vi "Load Settings from XML.vi"(8 "error in (no error)":errorcluster, 11 "Settings in":T1={"Hardware Configuration"={"AI"={"DAQmx Channel"="", "Max Input"=0.0, "Min Input"=0.0, "Sample Rate"=0.0, "DAQmx Task"="", "shunt resistor location"=-1, "external shunt resistor value"=249.0}, "AO"={"DAQmx Channel"="", "Max Output"=0.0, "Min Output"=0.0, "Sample Rate"=0.0, "DAQmx Task"=""}, "DO"={"DAQmx Channel"="", "Sample Rate"=0.0, "DAQmx Task"=""}, "DI"={"DAQmx Channel"="", "Sample Rate"=0.0, "DAQmx Task"=""}, "TC"={"DAQmx Channel"="", "Max Inout"=0.0, "Min Input"=0.0, "Sample Rate"=0.0, "DAQmx Task"="", "resistance configuration"=4, "r0"=100.0, "current excitation value"=0.0025, "current excitation source"=10167, "rtd type"=12481}}, "Logging Configuration"={"Log File Base Path"=path "", "TDMS File Reference"=refnum, "Samples to Save"=0, "Trigger - Time"=0, "Trigger - Threshold"=0.0, "Trigger - Channel"=0, "Enable Time Trigger"=FALSE, "Enable Threshold Trigger"=FALSE, "Always Log"=FALSE}} {"Hardware Configuration"."TC"."rtd type" items=["Pt3750"=12481, "Pt3851"=10071, "Pt3911"=12482, "Pt3916"=10069, "Pt3920"=10053, "Pt3928"=12483, "Custom"=10137]; "Hardware Configuration"."TC"."current excitation source" items=["Internal"=10200, "External"=10167, "None"=10230]; "Hardware Configuration"."TC"."resistance configuration" items=["2-Wire"=2, "3-Wire"=3, "4-Wire"=4]; "Hardware Configuration"."AI"."shunt resistor location" items=["default"=-1, "RSE"=10083, "NRSE"=10078, "Differential"=10106, "Pseudodifferential"=12529]}) -> (0 "error out":errorcluster, 3 "Settings out":T1={"Hardware Configuration"={"AI"={"DAQmx Channel"="", "Max Input"=0.0, "Min Input"=0.0, "Sample Rate"=0.0, "DAQmx Task"="", "shunt resistor location"=-1, "external shunt resistor value"=249.0}, "AO"={"DAQmx Channel"="", "Max Output"=0.0, "Min Output"=0.0, "Sample Rate"=0.0, "DAQmx Task"=""}, "DO"={"DAQmx Channel"="", "Sample Rate"=0.0, "DAQmx Task"=""}, "DI"={"DAQmx Channel"="", "Sample Rate"=0.0, "DAQmx Task"=""}, "TC"={"DAQmx Channel"="", "Max Inout"=0.0, "Min Input"=0.0, "Sample Rate"=0.0, "DAQmx Task"="", "resistance configuration"=4, "r0"=100.0, "current excitation value"=0.0025, "current excitation source"=10167, "rtd type"=12481}}, "Logging Configuration"={"Log File Base Path"=path "", "TDMS File Reference"=refnum, "Samples to Save"=0, "Trigger - Time"=0, "Trigger - Threshold"=0.0, "Trigger - Channel"=0, "Enable Time Trigger"=FALSE, "Enable Threshold Trigger"=FALSE, "Always Log"=FALSE}} {"Hardware Configuration"."TC"."rtd type" items=["Pt3750"=12481, "Pt3851"=10071, "Pt3911"=12482, "Pt3916"=10069, "Pt3920"=10053, "Pt3928"=12483, "Custom"=10137]; "Hardware Configuration"."TC"."current excitation source" items=["Internal"=10200, "External"=10167, "None"=10230]; "Hardware Configuration"."TC"."resistance configuration" items=["2-Wire"=2, "3-Wire"=3, "4-Wire"=4]; "Hardware Configuration"."AI"."shunt resistor location" items=["default"=-1, "RSE"=10083, "NRSE"=10078, "Differential"=10106, "Pseudodifferential"=12529]})   [LabVIEW 2024, in "Settings.lvlib"]
doc: "Attempts to load previous user specified settings from an XML file.\n\nThis VI will not generate an error. If a suitable XML file can't be loaded and parsed then it will simply return the default settings."
uses:
  Settings.lvlib
  Settings.ctl
  Acquisition/Hardware Configuration.ctl
  Logging/Logging Configuration.ctl
  <vilib>/Utility/xml.llb/Read From XML File(string).vi
  <vilib>/Utility/xml.llb/Write to XML File(string).vi
  Acquisition/Acquisition.lvlib
  Logging/Logging.lvlib
panel:
  # "(Scroll up for Settings Controls)"
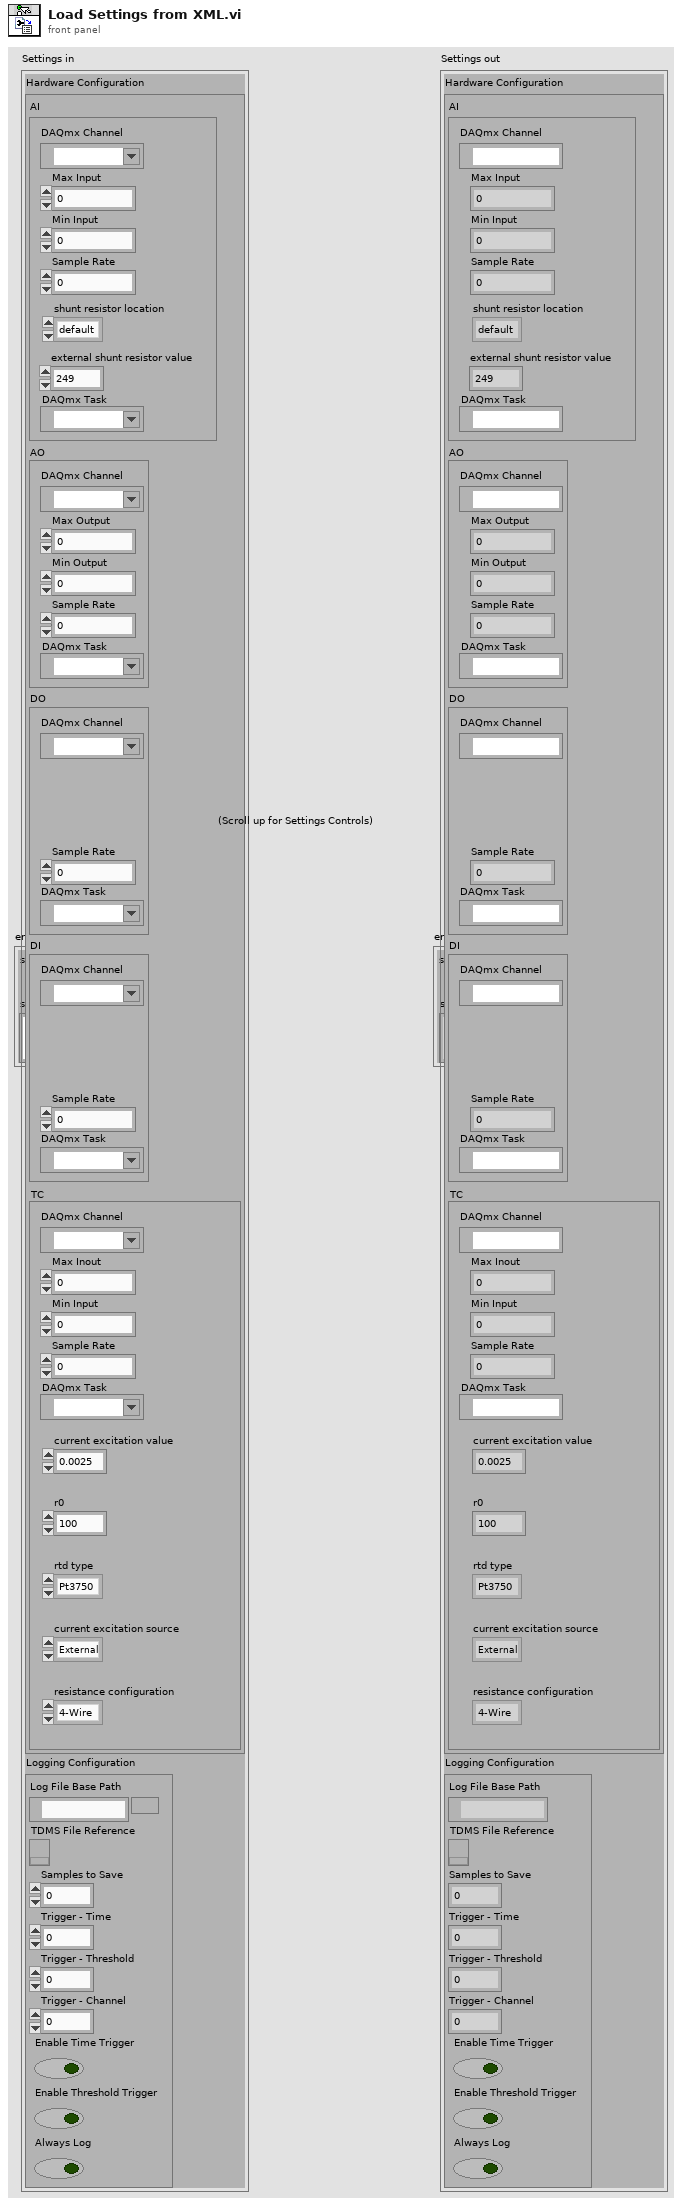
[diagram p1: front panel]
types:
  T1 = typedef "Settings.lvlib/Settings.ctl" = cluster{"Hardware Configuration":T2, "Logging Configuration":T3}
  T2 = typedef "Acquisition.lvlib/Hardware Configuration.ctl" = cluster{"AI":cluster{"DAQmx Channel":tag, "Max Input":dbl, "Min Input":dbl, "Sample Rate":dbl, "DAQmx Task":refnum<k21>, "shunt resistor location":i32, "external shunt resistor value":dbl}, "AO":cluster{"DAQmx Channel":tag, "Max Output":dbl, "Min Output":dbl, "Sample Rate":dbl, "DAQmx Task":refnum<k21>}, "DO":cluster{"DAQmx Channel":tag, "Sample Rate":dbl, "DAQmx Task":refnum<k21>}, "DI":cluster{"DAQmx Channel":tag, "Sample Rate":dbl, "DAQmx Task":refnum<k21>}, "TC":cluster{"DAQmx Channel":tag, "Max Inout":dbl, "Min Input":dbl, "Sample Rate":dbl, "DAQmx Task":refnum<k21>, "resistance configuration":i32, "r0":dbl, "current excitation value":dbl, "current excitation source":i32, "rtd type":i32}}
  T3 = typedef "Logging.lvlib/Logging Configuration.ctl" = cluster{"Log File Base Path":path, "TDMS File Reference":refnum<k34>, "Samples to Save":u32, "Trigger - Time":u32, "Trigger - Threshold":dbl, "Trigger - Channel":u32, "Enable Time Trigger":bool, "Enable Threshold Trigger":bool, "Always Log":bool}
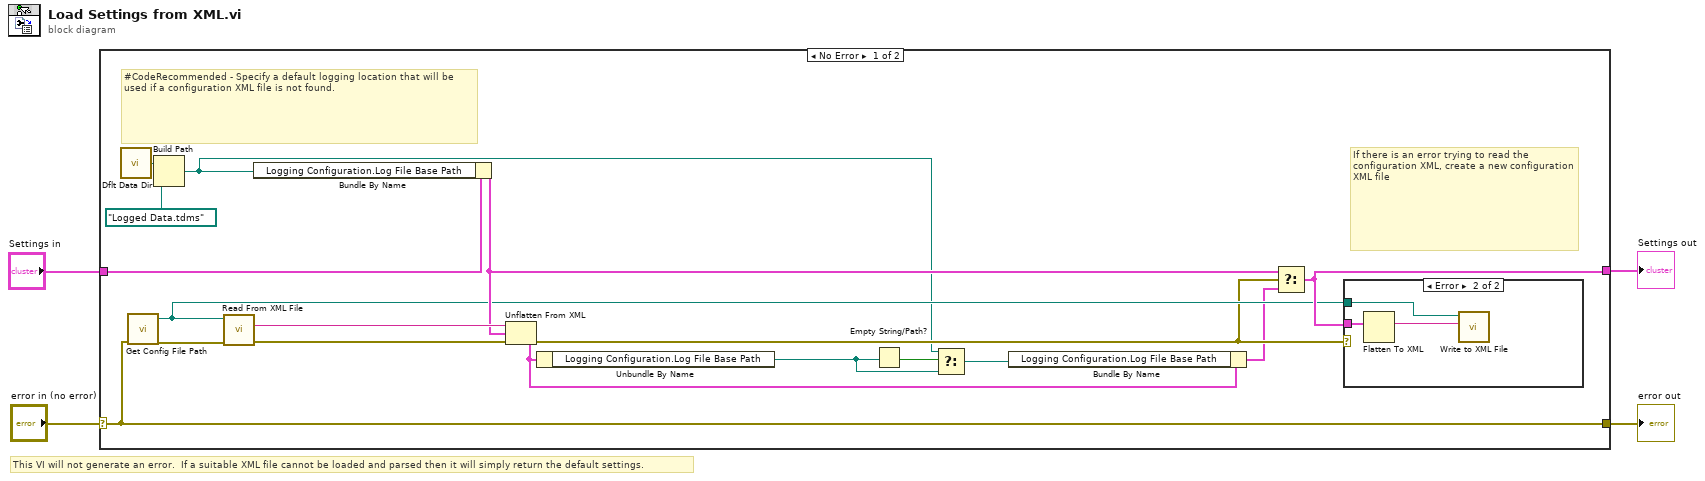
[diagram p0: block diagram]
diagram:
  # "This VI will not generate an error.  If a suitable XML file cannot be loaded and parsed then it will simply return the default settings."
  n1 = case shown="No Error" "error in (no error)" {
    selector: "error in (no error)" -> [w19 w26]
    tunnel: [w19 w26] -> w3
    tunnel: "Settings in" -> [w18 w25]
    tunnel: [w14 w25] -> w1
    frame No Error {
      # "If there is an error trying to read the configuration XML, create a new configuration XML file"
      # "#CodeRecommended - Specify a default logging location that will be used if a configuration XML file is not found."
      n2 = call <vilib>:"Dflt Data Dir.vi"() -> ("App:Default Data Directory"=w16:path)
      n3 = call "Get Config File Path.vi"("error in (no error)"=w19) -> ("error out"=w21:errorcluster, "XML File Path"=w13:path)  [unwired: 9 in]
      n4 = Build Path(base path=w16, name or relative path=path "Logged Data.tdms" ("App:Default Data Directory")) -> (appended path=w9:path)
      n5 = call-poly <vilib>:"Read From XML File.vi"("error in (no error)"=w21, "XML File Path"=w13) -> ("error out"=w12:errorcluster, "XML Elements"=w20:string)  [unwired: 7 in, 1 out]
      n6 = Bundle By Name(cluster=w18, "Logging Configuration.Log File Base Path"=w9) -> (w17:T1)
      n7 = Unflatten From XML(xml string=w20, type=w17, error in (no error)=w12) -> (value=w7:T1, error out=w11:errorcluster)
      n8 = Unbundle By Name(w7) -> ("Logging Configuration.Log File Base Path"=w5:path)
      n9 = Empty String/Path?(string/path=w5) -> (empty?=w10:bool)
      n10 = Select(t=w9, s=w10, f=w5) -> (s? t:f=w8:path)
      n11 = Bundle By Name(cluster=w7, "Logging Configuration.Log File Base Path"=w8) -> (w6:T1)
      n12 = Select(t=w17, s=w11, f=w6) -> (s? t:f=w14:T1)
      n13 = case shown="Error" w11 {
        tunnel: w14 -> [_ w24]
        tunnel: w13 -> [_ w22]
        frame No Error {
        }
        frame Error {
          n14 = Flatten To XML(6:w24) -> (2:w23:string)
          n15 = call-poly <vilib>:"Write to XML File.vi"("XML Input"=w23, "XML File Path"=w22) -> ()  [unwired: 7 in, 3 out]
        }
      }
    }
    frame Error {
    }
  }
  "error out" <- w3
  "Settings out" <- w1
